vi "Configure Pattern State Logic.vi"(5 "Clock Source (1: Channel 1)":i32(ring)=1 items=["Channel 1"=1, "Channel 2"=2, "Channel 3"=3, "Channel 4"=4, "Digital 0"=13, "Digital 1"=14, "Digital 2"=15, "Digital 3"=16, "Digital 4"=17, "Digital 5"=18, "Digital 6"=19, "Digital 7"=20, "Digital 8"=21, "Digital 9"=22, "Digital 10"=23, "Digital 11"=24, "Digital 12"=25, "Digital 13"=26, "Digital 14"=27, "Digital 15"=28], 7 "Enable Clock Source (False)":bool, 8 "Model":u32, 9 "Digital Channel Pattern":string, 10 "Analog Channel Pattern":string, 11 "Input":string) -> (0 "Output":string)   [LabVIEW 2012, in "Agilent 8000 Series.lvlib"]
doc: "Configures State/Pattern settings for an oscilloscope. It configures logic pattern to look for."
uses:
  <instrlib>/Agilent 8000 Series/Agilent 8000 Series.lvlib
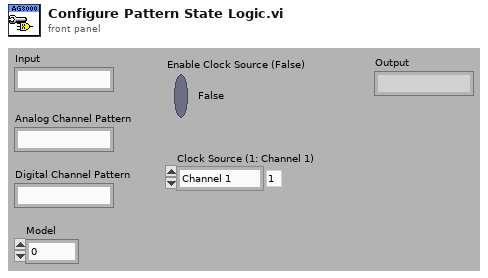
[diagram p1: front panel]
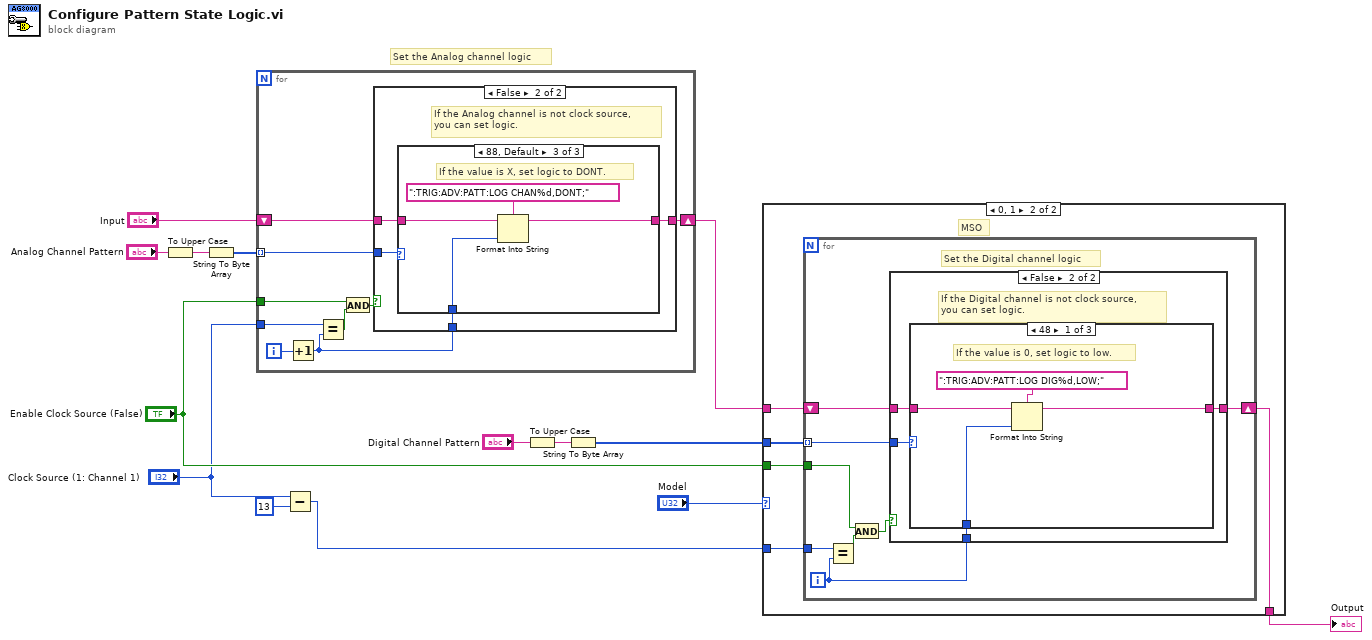
[diagram p0: block diagram]
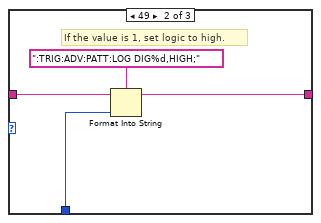
[diagram p4: hidden frame]
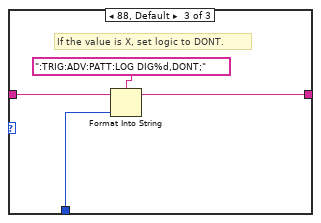
[diagram p5: hidden frame]
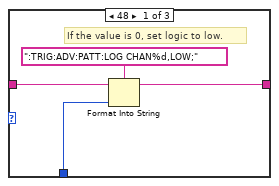
[diagram p7: hidden frame]
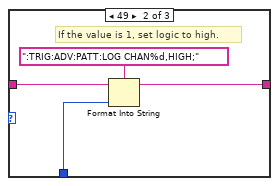
[diagram p8: hidden frame]
diagram:
  # "Set the Analog channel logic"
  n1 = To Upper Case(1:"Analog Channel Pattern") -> (0:w5:string)
  n2 = String To Byte Array(string=w5) -> (unsigned byte array=w6:u8[])
  n3 = for {
    tunnel: w6 -> [w23] mode=indexing
    shift-right: [w21] -> w13
    shift-left: "Input" -> [w22]
    tunnel: "Enable Clock Source (False)" -> [w19]
    tunnel: "Clock Source (1: Channel 1)" -> [w16]
    i -> [w20]
    n4 = Increment(x=w20) -> (x+1=w18:i32)
    n5 = Equal?(x=w16, y=w18) -> (x = y?=w17:bool)
    n6 = And(x=w19, y=w17) -> (x .and. y?=w15:bool)
    n7 = case shown="False" w15 {
      tunnel: w23 -> [_ w28]
      tunnel: w22 -> [w24 w27]
      tunnel: [w24 w26] -> w21
      tunnel: w18 -> [_ w25]
      frame True {
        # "If Analog Channel is Clock Source, \nit can not set logic."
      }
      frame False {
        # "If the Analog channel is not clock source,\nyou can set logic."
        n8 = case shown="88, Default" w28 {
          tunnel: w27 -> [w30 w35 w38]
          tunnel: w25 -> [w31 w33 w39]
          tunnel: [w29 w34 w37] -> w26
          frame 48 {
            # "If the value is 0, set logic to low."
            n9 = Format Into String(format string=":TRIG:ADV:PATT:LOG CHAN%d,LOW;", initial string=w30, w31) -> (resulting string=w29:string)  [unwired: 1 in, 1 out]
          }
          frame 49 {
            # "If the value is 1, set logic to high."
            n10 = Format Into String(format string=":TRIG:ADV:PATT:LOG CHAN%d,HIGH;", initial string=w35, w33) -> (resulting string=w34:string)  [unwired: 1 in, 1 out]
          }
          frame 88, Default {
            # "If the value is X, set logic to DONT."
            n11 = Format Into String(format string=":TRIG:ADV:PATT:LOG CHAN%d,DONT;", initial string=w38, w39) -> (resulting string=w37:string)  [unwired: 1 in, 1 out]
          }
        }
      }
    }
  }
  n12 = Subtract(x="Clock Source (1: Channel 1)", y=u16 13) -> (x-y=w1:i32)
  n13 = To Upper Case(1:"Digital Channel Pattern") -> (0:w10:string)
  n14 = String To Byte Array(string=w10) -> (unsigned byte array=w12:u8[])
  n15 = case shown="0, 1" "Model" {
    tunnel: w12 -> [_ w46]
    tunnel: w13 -> [w41 w45]
    tunnel: [w41 w44] -> w14
    tunnel: "Enable Clock Source (False)" -> [_ w43]
    tunnel: w1 -> [_ w42]
    frame Default {
      # "DSO"
    }
    frame 0, 1 {
      # "MSO"
      n16 = for {
        tunnel: w46 -> [w54] mode=indexing
        shift-right: [w52] -> w44
        shift-left: w45 -> [w53]
        tunnel: w43 -> [w51]
        tunnel: w42 -> [w49]
        i -> [w50]
        # "Set the Digital channel logic"
        n17 = Equal?(x=w49, y=w50) -> (x = y?=w48:bool)
        n18 = And(x=w51, y=w48) -> (x .and. y?=w47:bool)
        n19 = case shown="False" w47 {
          tunnel: w54 -> [_ w59]
          tunnel: w53 -> [w55 w58]
          tunnel: [w55 w57] -> w52
          tunnel: w50 -> [_ w56]
          frame True {
            # "If Digital Channel is Clock Source, \nit can not set logic."
          }
          frame False {
            # "If the Digital channel is not clock source,\nyou can set logic."
            n20 = case shown="48" w59 {
              tunnel: w58 -> [w61 w66 w69]
              tunnel: w56 -> [w62 w64 w70]
              tunnel: [w60 w65 w68] -> w57
              frame 48 {
                # "If the value is 0, set logic to low."
                n21 = Format Into String(format string=":TRIG:ADV:PATT:LOG DIG%d,LOW;", initial string=w61, w62) -> (resulting string=w60:string)  [unwired: 1 in, 1 out]
              }
              frame 49 {
                # "If the value is 1, set logic to high."
                n22 = Format Into String(format string=":TRIG:ADV:PATT:LOG DIG%d,HIGH;", initial string=w66, w64) -> (resulting string=w65:string)  [unwired: 1 in, 1 out]
              }
              frame 88, Default {
                # "If the value is X, set logic to DONT."
                n23 = Format Into String(format string=":TRIG:ADV:PATT:LOG DIG%d,DONT;", initial string=w69, w70) -> (resulting string=w68:string)  [unwired: 1 in, 1 out]
              }
            }
          }
        }
      }
    }
  }
  "Output" <- w14
